vi "ReconnectionProcedureArray.vi"(2 "Error In":errorcluster, 3 "Port Array":u16[](array[numeric]), 4 "TCP Array":refnum<k5>[](array[refnum])) -> (0 "Error Out":errorcluster, 1 "TCP Array 2":refnum<k5>[](array[refnum]))   [LabVIEW 2014]
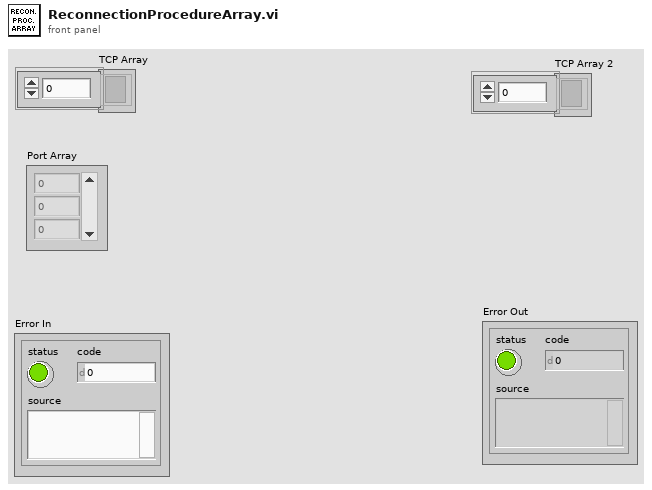
[diagram p1: front panel]
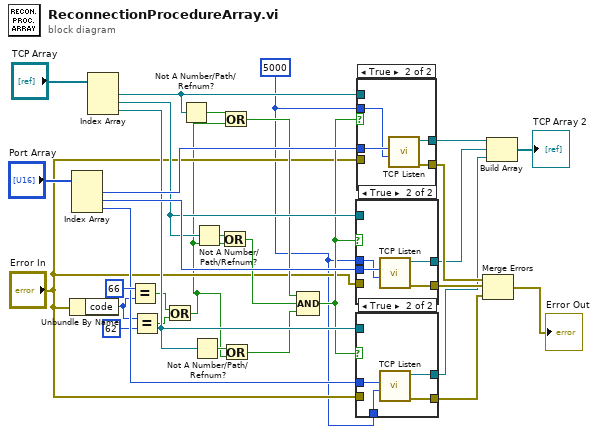
[diagram p0: block diagram]
diagram:
  w1 = 5000
  n1 = Unbundle By Name("Error In") -> ("code"=w6:i32)
  n2 = Index Array(array="Port Array") -> (element #1=w28:u16, element #2=w25:u16, element #3=w24:u16)  [unwired: 3 in]
  n3 = Index Array(array="TCP Array") -> (element #1=w26:refnum<k5>, element #2=w21:refnum<k5>, element #3=w20:refnum<k5>)  [unwired: 3 in]
  n4 = Equal?(x=66, y=w6) -> (x = y?=w4:bool)
  n5 = Equal?(x=w6, y=62) -> (x = y?=w5:bool)
  n6 = Or(x=w4, y=w5) -> (x .or. y?=w3:bool)
  n7 = Not A Number/Path/Refnum?(number/path/refnum=w26) -> (NaN/Path/Refnum?=w31:bool)
  n8 = Not A Number/Path/Refnum?(number/path/refnum=w20) -> (NaN/Path/Refnum?=w22:bool)
  n9 = Not A Number/Path/Refnum?(number/path/refnum=w21) -> (NaN/Path/Refnum?=w23:bool)
  n10 = Or(x=w23, y=w3) -> (x .or. y?=w18:bool)
  n11 = Or(x=w31, y=w3) -> (x .or. y?=w19:bool)
  n12 = Or(x=w22, y=w3) -> (x .or. y?=w17:bool)
  n13 = Compound Arithmetic op=AND(w19, w18, w17) -> (w16:bool)
  n14 = case shown="True" w16 {
    tunnel: [w33 w37] -> w9
    tunnel: w21 -> [w33 _]
    tunnel: w25 -> [_ w36]
    tunnel: [w32 w35] -> w13
    tunnel: "Error In" -> [w32 _]
    tunnel: w1 -> [_ w34]
    frame False {
    }
    frame True {
      n15 = call <vilib>:"TCP Listen.vi"("timeout ms (wait forever: -1)"=w34, "port"=w36) -> ("error out"=w35:errorcluster, "connection ID"=w37:refnum<k5>)  [unwired: 5 in, 3 out]
    }
  }
  n16 = case shown="True" w16 {
    tunnel: [w39 w43] -> w8
    tunnel: w20 -> [w39 _]
    tunnel: w24 -> [_ w42]
    tunnel: [w38 w41] -> w12
    tunnel: "Error In" -> [w38 _]
    tunnel: w1 -> [_ w40]
    frame False {
    }
    frame True {
      n17 = call <vilib>:"TCP Listen.vi"("timeout ms (wait forever: -1)"=w40, "port"=w42) -> ("error out"=w41:errorcluster, "connection ID"=w43:refnum<k5>)  [unwired: 5 in, 3 out]
    }
  }
  n18 = case shown="True" w16 {
    tunnel: w28 -> [_ w49]
    tunnel: [w45 w48] -> w10
    tunnel: w26 -> [w45 _]
    tunnel: [w44 w47] -> w14
    tunnel: "Error In" -> [w44 _]
    tunnel: w1 -> [_ w46]
    frame False {
    }
    frame True {
      n19 = call <vilib>:"TCP Listen.vi"("timeout ms (wait forever: -1)"=w46, "port"=w49) -> ("error out"=w47:errorcluster, "connection ID"=w48:refnum<k5>)  [unwired: 5 in, 3 out]
    }
  }
  n20 = Merge Errors(w14, w13, w12) -> (→"Error Out":errorcluster)
  n21 = Build Array(w10, w9, w8) -> (→"TCP Array 2":refnum<k5>[])
